vi "EnviarParametros_MOVIMIENTOABS.vi"(0 "VISA resource name":refnum<visa-resource-name>, 1 "PASOS EN X":i32, 2 "PASOS EN Y":i32, 3 "PASOS EN Z":i32, 5 "error in (no error)":errorcluster) -> (14 "VISA resource name 2":refnum<visa-resource-name>, 17 "read buffer":string, 18 "enviados":string, 19 "error IO":errorcluster)   [LabVIEW 2019]
uses:
  <vilib>/Utility/error.llb/Error Cluster From Error Code.vi
  <vilib>/ErrorRing/Error Ring.xnode
panel:
  out "return count 2":u32
  out "return count":u32
  out "Parametros enviados = Parametros leídos?":bool
  # "/* Teoricamente:\n1mm= 91 pasos\n1cm = 910 pasos\n10 cm = 9100 pasos\n0.1 mm = 9 pasos aprox\n*/"
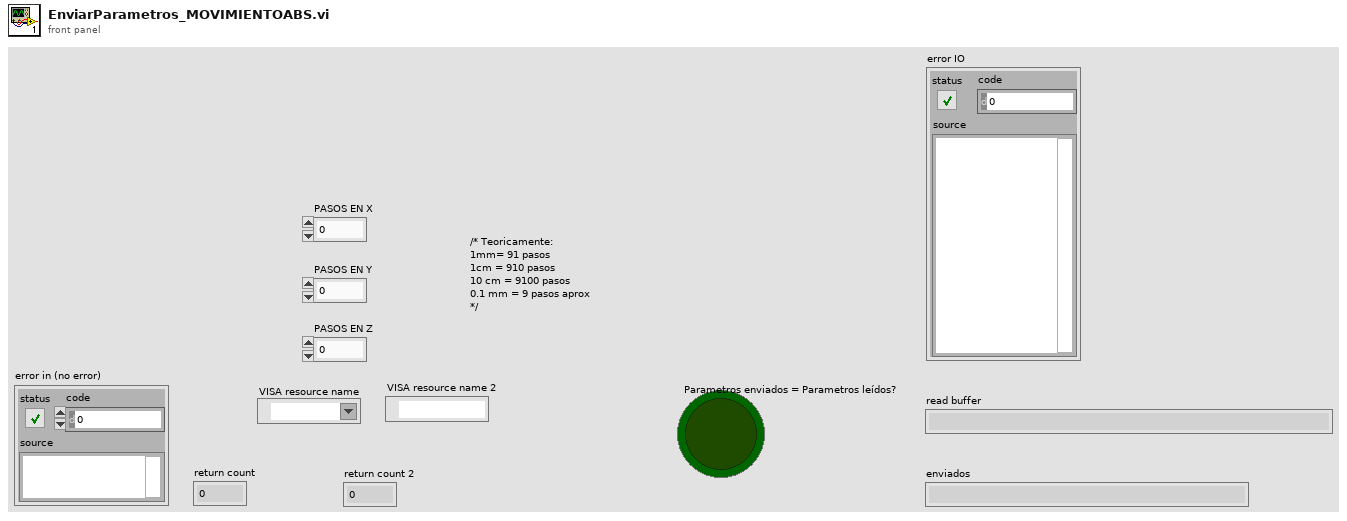
[diagram p1: front panel]
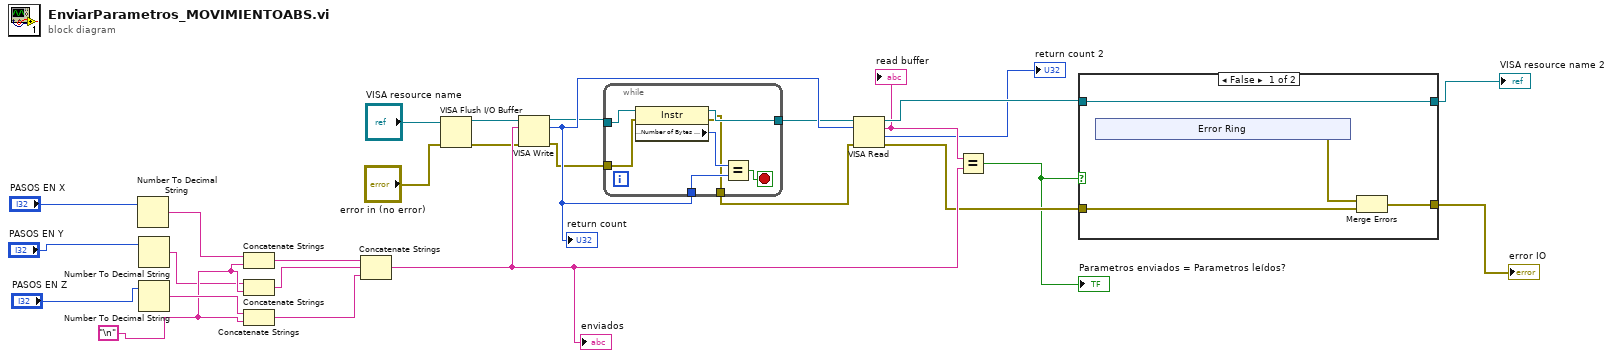
[diagram p0: block diagram]
diagram:
  w15 = "\n"
  n1 = Number To Decimal String(number="PASOS EN X") -> (decimal integer string=w13:string)  [unwired: 1 in]
  n2 = Number To Decimal String(number="PASOS EN Y") -> (decimal integer string=w14:string)  [unwired: 1 in]
  n3 = Number To Decimal String(number="PASOS EN Z") -> (decimal integer string=w17:string)  [unwired: 1 in]
  n4 = Concatenate Strings(w13, w15) -> (w19:string)
  n5 = Concatenate Strings(w14, w15) -> (w18:string)
  n6 = Concatenate Strings(w17, w15) -> (w16:string)
  n7 = Concatenate Strings(w19, w18, w16) -> (w25:string)
  "enviados" <- w25
  n8 = VISA Flush I/O Buffer(VISA resource name="VISA resource name", error in (no error)="error in (no error)") -> (VISA resource name out=w10:refnum<visa-resource-name>, error out=w11:errorcluster)  [unwired: 1 in]
  n9 = VISA Write(VISA resource name=w10, write buffer=w25, error in (no error)=w11) -> (VISA resource name out=w7:refnum<visa-resource-name>, return count=w8:u32, error out=w5:errorcluster)
  "return count" <- w8
  n10 = while {
    tunnel: w8 -> [w33]
    tunnel: w7 -> [w31]
    tunnel: [w30] -> w6
    tunnel: w5 -> [w29]
    tunnel: [w28] -> w4
    stop <- w32 stop-if-true
    n11 = property class="Instr"(reference=w31, error in=w29) -> (reference out=w30:refnum<visa-resource-name>, error out=w28:errorcluster, "Serial Settings:Number of Bytes at Serial Port"=w34:u32)
    n12 = Equal?(x=w34, y=w33) -> (x = y?=w32:bool)
  }
  n13 = VISA Read(VISA resource name=w6, byte count=w8, error in (no error)=w4) -> (VISA resource name out=w22:refnum<visa-resource-name>, read buffer=w12:string, return count=→"return count 2":u32, error out=w24:errorcluster)
  "read buffer" <- w12
  n14 = Equal?(x=w12, y=w25) -> (x = y?=w20:bool)
  "Parametros enviados = Parametros leídos?" <- w20
  n15 = case shown="False" w20 {
    tunnel: w24 -> [w37 w44]
    tunnel: [w36 w44] -> w23
    tunnel: w22 -> [w35 w45]
    tunnel: [w35 w45] -> w21
    frame False {
      n16 = xnode "Error Ring"() -> ("error out"=w38:errorcluster)
      n17 = Merge Errors(w38, w37) -> (w36:errorcluster)
    }
    frame True {
    }
  }
  "error IO" <- w23
  "VISA resource name 2" <- w21
